vi "f_OFF_Region.vi"(0 "VISA Resource Name":refnum<visa-resource-name>, 1 "Project #":string, 2 "Request #":string, 3 "TEST #":string, 4 "ICE":dbl, 5 "VGE":dbl, 6 "VCE":dbl, 7 "error in (no error)":errorcluster) -> (8 "Tdoff (ns)":dbl, 9 "Di (A)":dbl, 10 "Tf (ns)":dbl, 11 "Dt (ns)":dbl, 12 "Di/Dt (A/us)":dbl, 14 "Dv/Dt (V/us)":dbl, 16 "Eoff (uj)":dbl, 17 "Dv (V)":dbl, 19 "Dt (ns) 2":dbl, 20 "DONE Tdoff":bool, 21 "DONE Tf":bool, 22 "DONE Di/Dt OFF":bool, 23 "DONE Dv/Dt OFF":bool, 24 "DONE Eoff":bool, 27 "error out":errorcluster)   [LabVIEW 2020]
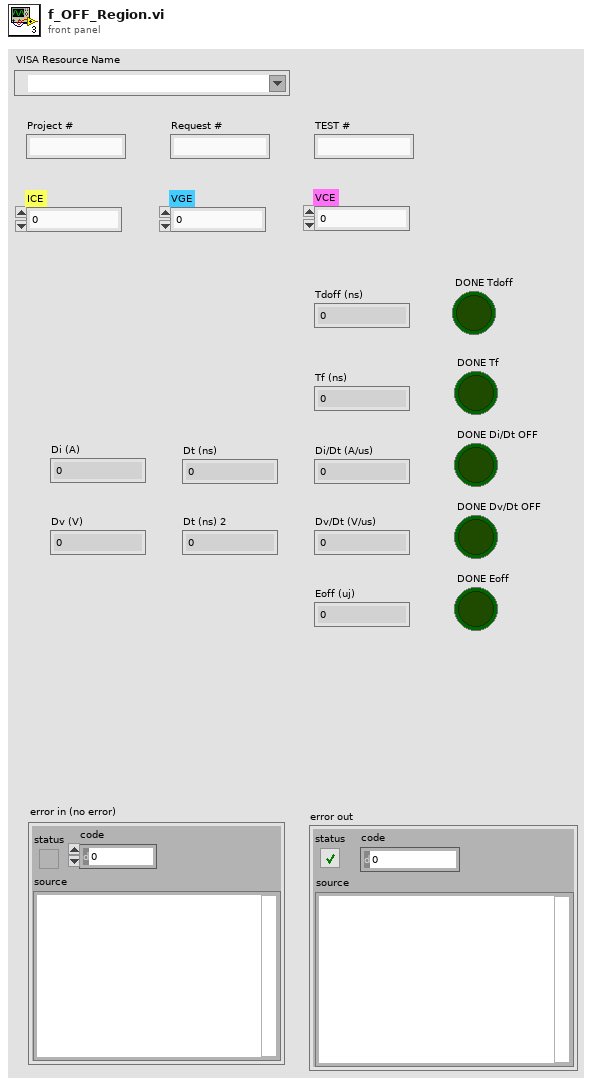
[diagram p1: front panel]
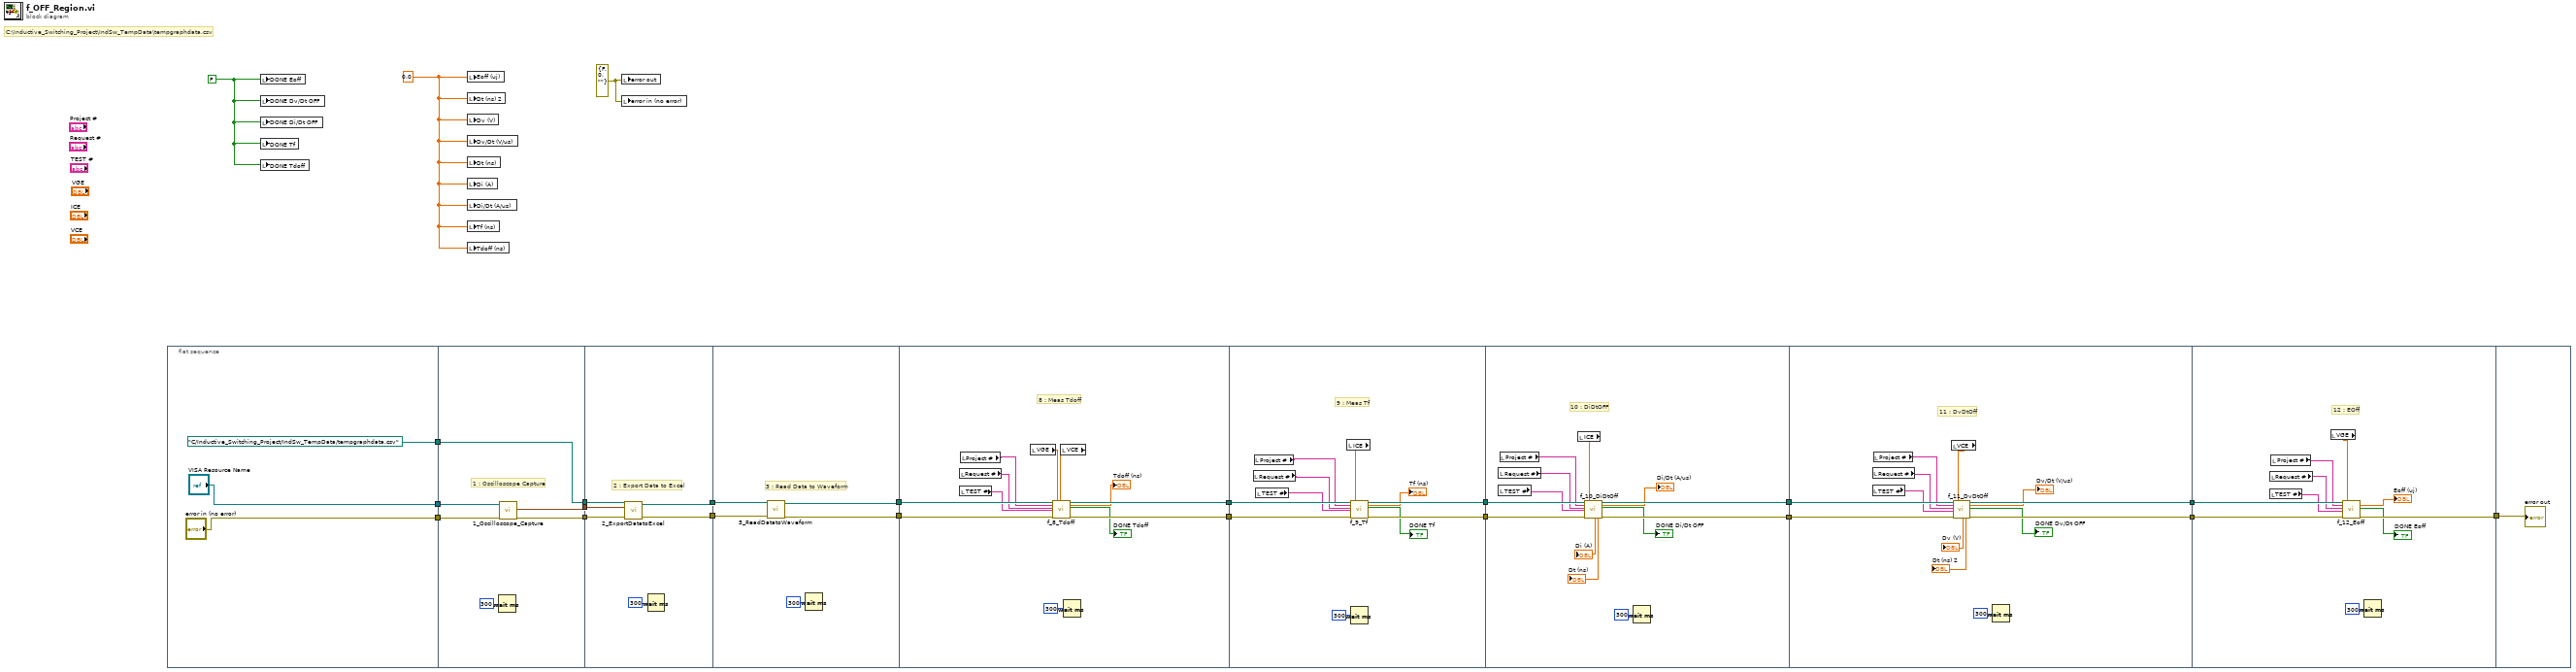
[diagram p0: block diagram]
diagram:
  w1 = errorcluster {"status"=FALSE, "code"=0, "source"=""} ("error out")
  w2 = 0.0 ("Eoff (uj)")
  w3 = FALSE ("DONE Eoff")
  # "C:\\Inductive_Switching_Project\\IndSw_TempData\\tempgraphdata.csv"
  n1 = flat-sequence {
    tunnel: [path "C:/Inductive_Switching_Project/IndSw_TempData/tempgraphdata.csv" ("file path (IN)")] -> w22
    tunnel: ["error in (no error)"] -> w21
    tunnel: ["VISA Resource Name"] -> w20
    tunnel: [w27] -> w19
    tunnel: [w26] -> w18
    tunnel: [w31] -> w17
    tunnel: w22 -> [w31]
    tunnel: w21 -> [w29]
    tunnel: w20 -> [w28]
    tunnel: [w33] -> w16
    tunnel: [w32] -> w15
    tunnel: w19 -> [w36]
    tunnel: w18 -> [w35]
    tunnel: w17 -> [w34]
    tunnel: [w38] -> w14
    tunnel: [w39] -> w13
    tunnel: w16 -> [w41]
    tunnel: w15 -> [w40]
    tunnel: [w50] -> w12
    tunnel: [w52] -> w11
    tunnel: w14 -> [w51]
    tunnel: w13 -> [w53]
    tunnel: [w61] -> w10
    tunnel: [w63] -> w9
    tunnel: w12 -> [w62]
    tunnel: w11 -> [w64]
    tunnel: [w74] -> w8
    tunnel: [w76] -> w7
    tunnel: w10 -> [w75]
    tunnel: w9 -> [w77]
    tunnel: [w89] -> w6
    tunnel: [w87] -> w5
    tunnel: w8 -> [w90]
    tunnel: w7 -> [w88]
    tunnel: [w99] -> w4
    tunnel: w6 -> [w98]
    tunnel: w5 -> [w100]
    tunnel: w4 -> [w102]
    frame #0 {
    }
    frame #1 {
      # "1 : Oscilloscope Capture"
      n2 = Wait (ms)(milliseconds to wait=u32 300) -> ()  [unwired: 1 out]
      n3 = call "1_Oscilloscope_Capture.vi"("error in (no error)"=w29, "VISA Resource Name"=w28) -> ("error out"=w27:errorcluster, "Waveform Graph"=w26:waveform(dbl)[])  [unwired: 7 in, 1 out]
    }
    frame #2 {
      # "2 : Export Data to Excel"
      n4 = call "2_ExportDatatoExcel.vi"("error in (no error)"=w36, "Waveform Graph"=w35, "file path (IN)"=w34) -> ("error out"=w33:errorcluster, "file path (OUT)"=w32:path)  [unwired: 7 in]
      n5 = Wait (ms)(milliseconds to wait=u32 300) -> ()  [unwired: 1 out]
    }
    frame #3 {
      # "3 : Read Data to Waveform"
      n6 = call "3_ReadDatatoWaveform.vi"("error in (no error)"=w41, "file path (IN)"=w40) -> ("error out"=w39:errorcluster, "file path (OUT)"=w38:path)  [unwired: 3 in, 5 out]
      n7 = Wait (ms)(milliseconds to wait=u32 300) -> ()  [unwired: 1 out]
    }
    frame #4 {
      # "8 : Meas Tdoff"
      n8 = local read "Request #"() -> (w48:string)
      n9 = local read "TEST #"() -> (w47:string)
      n10 = local read "Project #"() -> (w49:string)
      n11 = local read "VGE"() -> (w46:dbl)
      n12 = local read "VCE"() -> (w45:dbl)
      n13 = call "f_8_Tdoff.vi"("file path (IN)"=w51, "Project #"=w49, "Request #"=w48, "TEST #"=w47, "error in (no error)"=w53, "VGE"=w46, "VCE"=w45) -> ("file path (OUT)"=w50:path, "Tdoff (ns)"=→"Tdoff (ns)":dbl, "DONE Tdoff"=→"DONE Tdoff":bool, "error out"=w52:errorcluster)  [unwired: 9 in]
      n14 = Wait (ms)(milliseconds to wait=u32 300) -> ()  [unwired: 1 out]
    }
    frame #5 {
      # "9 : Meas Tf"
      n15 = local read "Request #"() -> (w59:string)
      n16 = local read "Project #"() -> (w60:string)
      n17 = local read "TEST #"() -> (w58:string)
      n18 = local read "ICE"() -> (w57:dbl)
      n19 = call "f_9_Tf.vi"("file path (IN)"=w62, "Project #"=w60, "Request #"=w59, "TEST #"=w58, "error in (no error)"=w64, "ICE"=w57) -> ("file path (OUT)"=w61:path, "Tf (ns)"=→"Tf (ns)":dbl, "DONE Tf"=→"DONE Tf":bool, "error out"=w63:errorcluster)  [unwired: 10 in]
      n20 = Wait (ms)(milliseconds to wait=u32 300) -> ()  [unwired: 1 out]
    }
    frame #6 {
      # "10 : DiDtOFF"
      n21 = local read "Request #"() -> (w72:string)
      n22 = local read "TEST #"() -> (w71:string)
      n23 = local read "Project #"() -> (w73:string)
      n24 = local read "ICE"() -> (w70:dbl)
      n25 = call "f_10_DiDtOff.vi"("file path (IN)"=w75, "Project #"=w73, "Request #"=w72, "TEST #"=w71, "error in (no error)"=w77, "ICE"=w70) -> ("Di (A)"=→"Di (A)":dbl, "Dt (ns)"=→"Dt (ns)":dbl, "file path (OUT)"=w74:path, "Di/Dt (A/us)"=→"Di/Dt (A/us)":dbl, "DONE Di/Dt OFF"=→"DONE Di/Dt OFF":bool, "error out"=w76:errorcluster)  [unwired: 8 in]
      n26 = Wait (ms)(milliseconds to wait=u32 300) -> ()  [unwired: 1 out]
    }
    frame #7 {
      # "11 : DvDtOff"
      n27 = local read "Request #"() -> (w85:string)
      n28 = local read "TEST #"() -> (w84:string)
      n29 = local read "Project #"() -> (w86:string)
      n30 = local read "VCE"() -> (w83:dbl)
      n31 = call "f_11_DvDtOff.vi"("file path (IN)"=w90, "Project #"=w86, "Request #"=w85, "TEST #"=w84, "error in (no error)"=w88, "VCE"=w83) -> ("Dv (V)"=→"Dv (V)":dbl, "Dt (ns)"=→"Dt (ns) 2":dbl, "file path (OUT)"=w89:path, "Dv/Dt (V/us)"=→"Dv/Dt (V/us)":dbl, "DONE Dv/Dt OFF"=→"DONE Dv/Dt OFF":bool, "error out"=w87:errorcluster)  [unwired: 8 in]
      n32 = Wait (ms)(milliseconds to wait=u32 300) -> ()  [unwired: 1 out]
    }
    frame #8 {
      # "12 : EOff"
      n33 = local read "Request #"() -> (w96:string)
      n34 = local read "TEST #"() -> (w95:string)
      n35 = local read "Project #"() -> (w97:string)
      n36 = local read "VGE"() -> (w94:dbl)
      n37 = call "f_12_Eoff.vi"("file path (IN)"=w98, "Project #"=w97, "Request #"=w96, "TEST #"=w95, "error in (no error)"=w100, "VGE"=w94) -> ("Eoff (uj)"=→"Eoff (uj)":dbl, "DONE Eoff"=→"DONE Eoff":bool, "error out"=w99:errorcluster)  [unwired: 10 in, 1 out]
      n38 = Wait (ms)(milliseconds to wait=u32 300) -> ()  [unwired: 1 out]
    }
    frame #9 {
      "error out" <- w102
    }
  }
  n39 = local write "DONE Eoff"(w3) -> ()
  n40 = local write "DONE Dv/Dt OFF"(w3) -> ()
  n41 = local write "DONE Di/Dt OFF"(w3) -> ()
  n42 = local write "DONE Tf"(w3) -> ()
  n43 = local write "DONE Tdoff"(w3) -> ()
  n44 = local write "Eoff (uj)"(w2) -> ()
  n45 = local write "Dt (ns) 2"(w2) -> ()
  n46 = local write "Dv (V)"(w2) -> ()
  n47 = local write "Dv/Dt (V/us)"(w2) -> ()
  n48 = local write "Dt (ns)"(w2) -> ()
  n49 = local write "Di (A)"(w2) -> ()
  n50 = local write "Di/Dt (A/us)"(w2) -> ()
  n51 = local write "Tf (ns)"(w2) -> ()
  n52 = local write "Tdoff (ns)"(w2) -> ()
  n53 = local write "error out"(w1) -> ()
  n54 = local write "error in (no error)"(w1) -> ()
